vi "gaussianFitTestWithData.vi"() -> ()   [LabVIEW 2017]
uses:
  <vilib>/Utility/file.llb/Read Delimited Spreadsheet (DBL).vi
panel:
  in  "nZ":i32=21
  out "x0":dbl[](array[numeric])
  out "x0,sigma,bg,amplitude":dbl[](array[numeric])
  out "XY Graph":cluster{dbl[], "z profile":dbl[]}[](graph)
  in  "index":i32
  # "0. Insert index of volume (z step of etl1) that you want to refit.\n1. Select single volume .dat file with frames\n2. Select single volume details file\n3. In the VI that opens, select a rectangle around the spot.\n4. Substitute the fitted value of x0 (in the array on the right) in the file\n    objectiveRegistrationRawZ.txt (second line, i-th entry)"
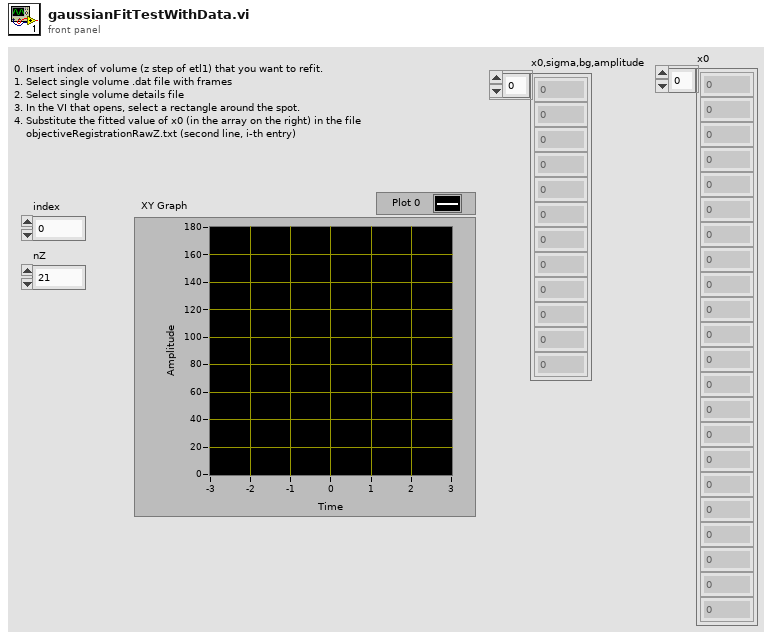
[diagram p1: front panel]
types:
  T1 = cluster{"positions (z)":dbl[], "z profile":dbl[]}
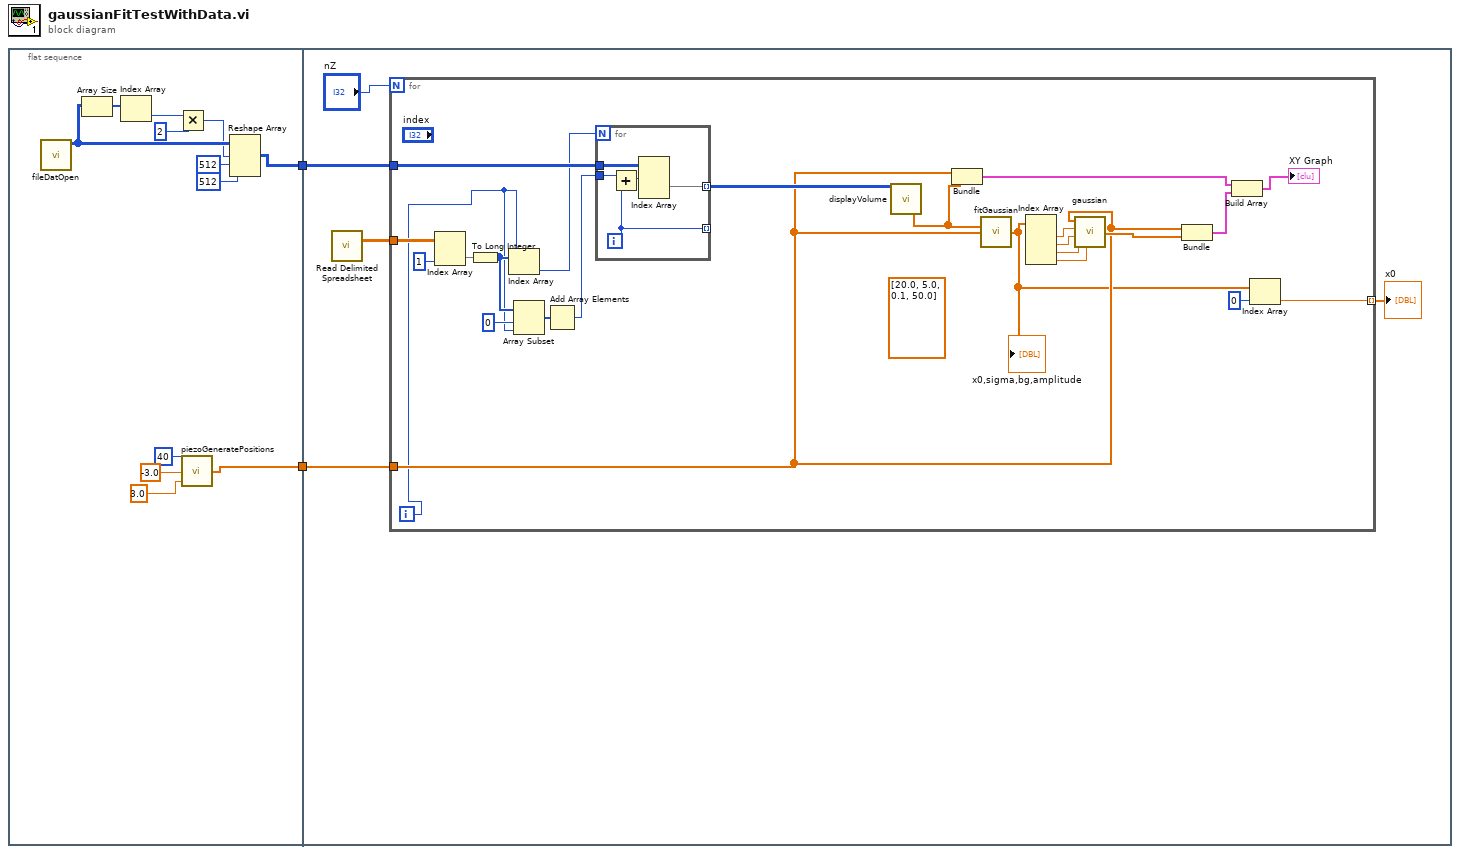
[diagram p0: block diagram]
diagram:
  n1 = flat-sequence {
    tunnel: [w10] -> w2
    tunnel: [w3] -> w1
    tunnel: w2 -> [w18]
    tunnel: w1 -> [w17]
    frame #0 {
      n2 = call "fileDatOpen.vi"() -> ("output array"=w13:u16[][][])  [unwired: 4 in, 3 out]
      n3 = Array Size(array=w13) -> (size(s)=w14:i32[])
      n4 = Index Array(array=w14) -> (element=w9:i32)  [unwired: 1 in]
      n5 = Multiply(x=w9, y=2) -> (x*y=w7:i32)
      n6 = call "piezoGeneratePositions.vi"("zf"=3.0, "z0"=-3.0, "M"=40) -> ("positions (z)"=w3:dbl[])
      n7 = Reshape Array(w13, w7, 512 ("dimension size"), 512 ("dimension size")) -> (w10:u16[][][])
    }
    frame #1 {
      n8 = call-poly <vilib>:"Read Delimited Spreadsheet.vi"() -> ("all rows"=w19:dbl[][])  [unwired: 10 in, 5 out]
      n9 = for {
        N: "nZ" -> [_]
        tunnel: w19 -> [w42]
        tunnel: w18 -> [w35]
        tunnel: w17 -> [w25]
        tunnel: [w20] -> w16 mode=indexing
        i -> [w23]
        (unwired) dbl[] [20.0, 5.0, 0.1, 50.0] ("initial parameters")
        n10 = Index Array(array=w42, index (col)=1 ("disabled index (col)")) -> (element=w41:dbl[])  [unwired: 1 in]
        n11 = To Long Integer(number=w41) -> (32bit integer=w39:i32[])
        n12 = Index Array(array=w39, index=w23) -> (element=w26:i32)
        n13 = Array Subset(array=w39, index=0, length=w23) -> (w37:i32[])
        n14 = Add Array Elements(numeric array=w37) -> (sum=w36:i32)
        n15 = for {
          N: w26 -> [_]
          tunnel: w35 -> [w48]
          tunnel: [w46] -> w40 mode=indexing
          tunnel: w36 -> [w45]
          tunnel: [w44] -> _ mode=indexing
          i -> [w44]
          n16 = Add(x=w45, y=w44) -> (x+y=w47:i32)
          n17 = Index Array(array=w48, index (dim 0)=w47) -> (element=w46:u16[][])  [unwired: 2 in]
        }
        n18 = call "displayVolume.vi"("frames"=w40) -> ("z profile"=w31:dbl[])  [unwired: 13 in, 5 out]
        n19 = Bundle("positions (z)"=w25, "z profile"=w31) -> (w30:T1)  [unwired: 1 in]
        n20 = call "fitGaussian.vi"("X"=w25, "Y"=w31) -> ("x0,sigma,bg,amplitude"=w22:dbl[])  [unwired: 1 in]
        "x0,sigma,bg,amplitude" <- w22
        n21 = Index Array(array=w22) -> (element #1=w34:dbl, element #2=w33:dbl, element #3=w32:dbl, element #4=w27:dbl)  [unwired: 4 in]
        n22 = call "gaussian.vi"("X"=w25, "x0"=w34, "sigma"=w33, "bg"=w32, "amplitude"=w27) -> ("Y"=w28:dbl[])
        n23 = Bundle("positions (z)"=w25, "Y"=w28) -> (w24:cluster{"positions (z)":dbl[], "Y":dbl[]})  [unwired: 1 in]
        n24 = Build Array(w30, w24) -> (→"XY Graph":cluster{"positions (z)":dbl[], "Y":dbl[]}[])
        n25 = Index Array(array=w22, index=0) -> (element=w20:dbl)
      }
      "x0" <- w16
    }
  }
